vi "System.vi"() -> ()   [LabVIEW 2020]
doc: "Use this template to build a producer/consumer design pattern with events to produce queue items. Use this design pattern instead of the User Interface Event Handler pattern for user interfaces when you want to execute code asynchronously in response to an event without slowing the user interface responsiveness."
uses:
  <vilib>/Instr/_visa.llb/VISA Configure Serial Port (Instr).vi
panel:
  in  "Initialize":bool
  out "Geneator Torque":dbl(knob) scale=0.0..10.0
  out "Generator Speed":dbl(knob) scale=0.0..100.0
  out "Motor Speed":dbl(knob) scale=0.0..100.0
  out "Motor Torque":dbl(knob) scale=0.0..10.0
  out "Motor Load":dbl(slide) scale=0.0..10.0
  out "PWM":dbl
  out "Data Read":string
  in  "Baud rate (9600)":u32=9600
  in  "Write Data":bool
  in  "Data PostFix":string
  in  "VISA resource name":refnum<visa-resource-name>
  in  "Close":bool
  in  "Open":bool
  out "Connected":bool
  in  "stop":bool
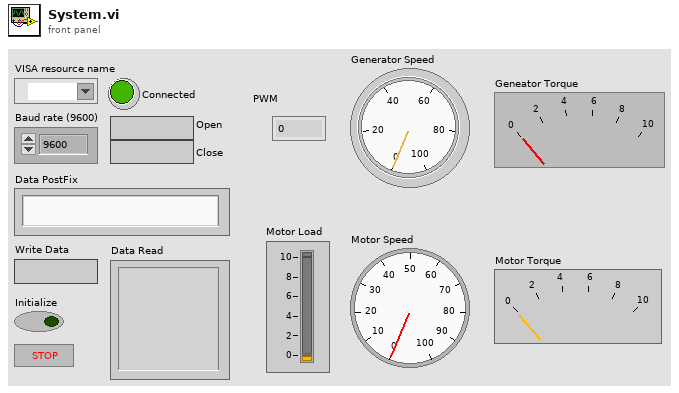
[diagram p1: front panel]
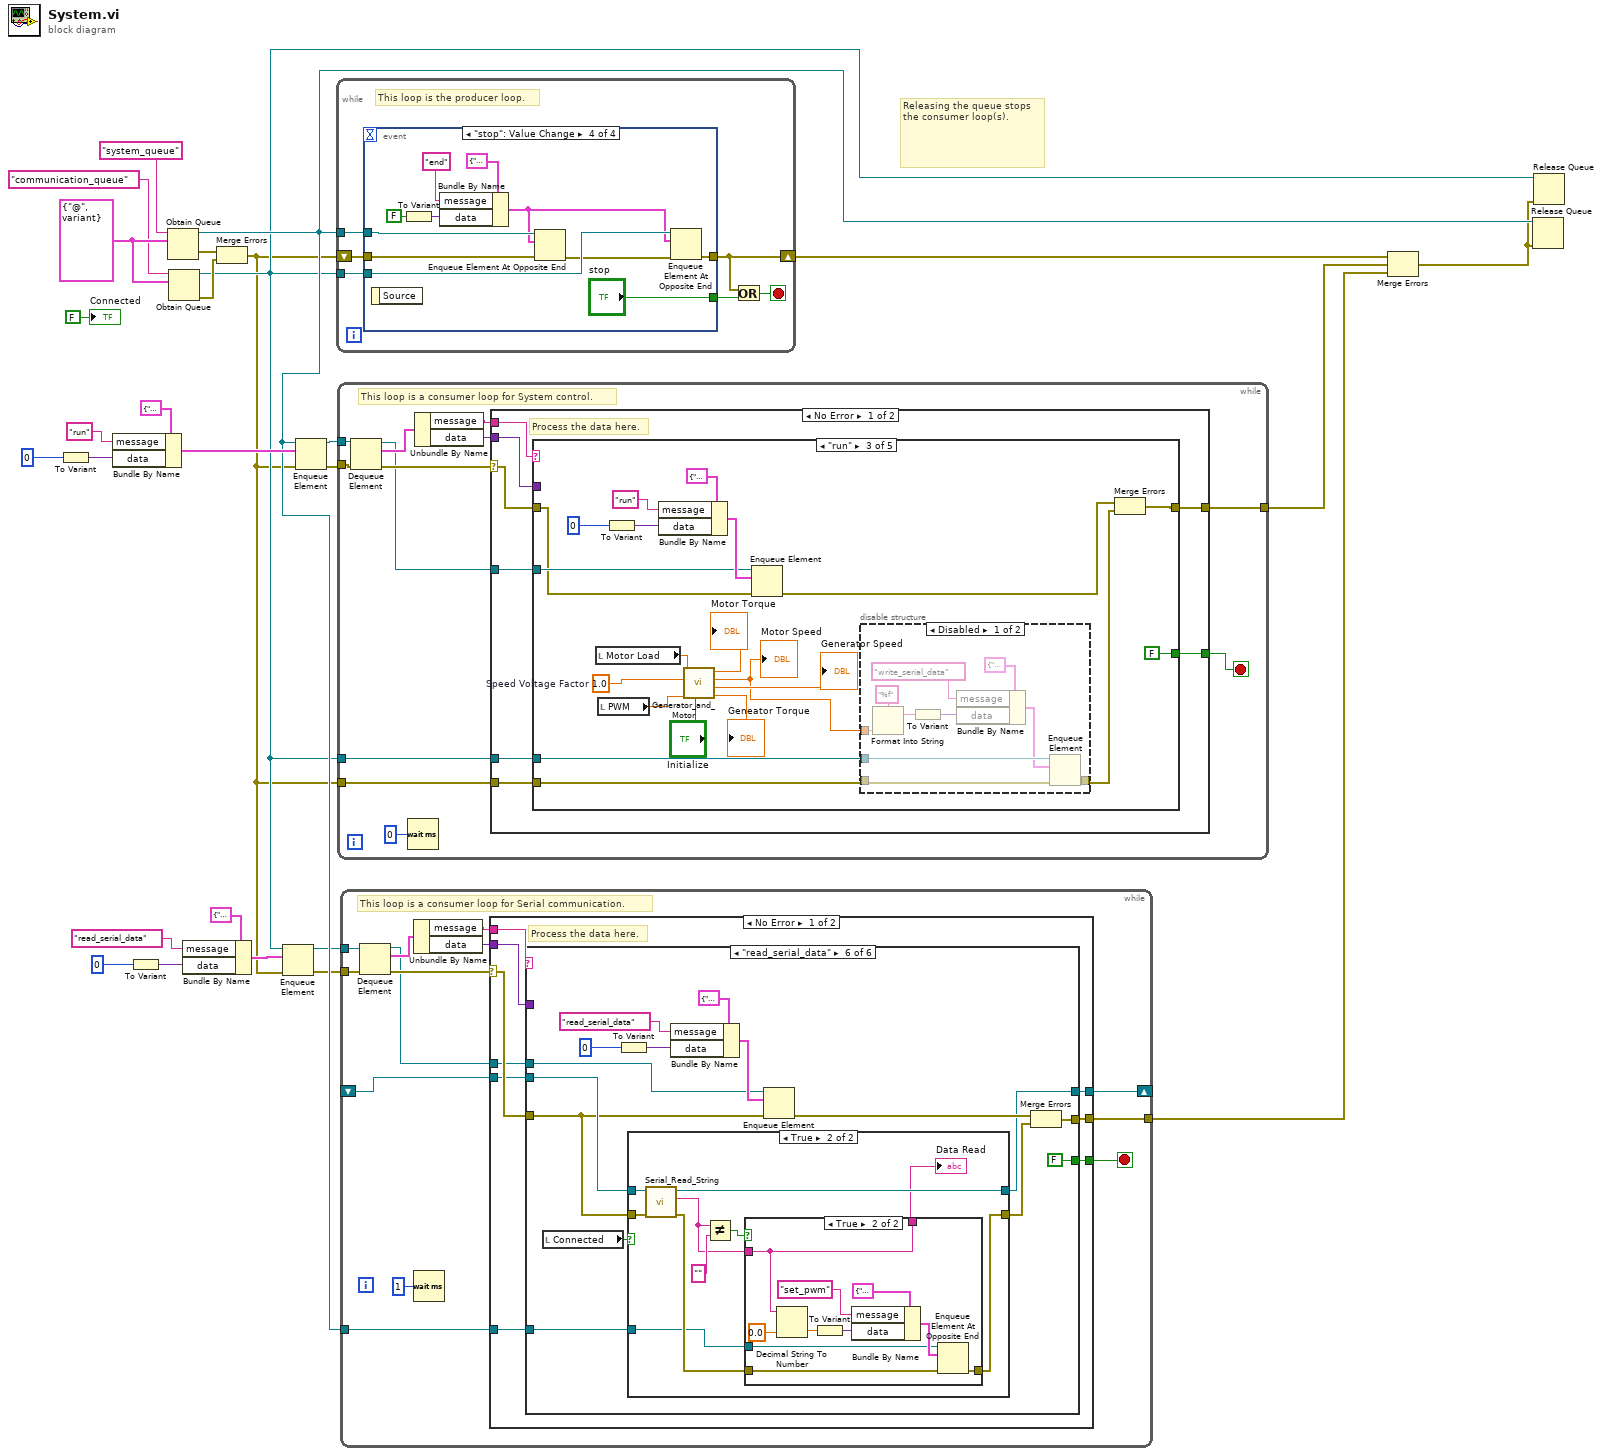
[diagram p0: block diagram]
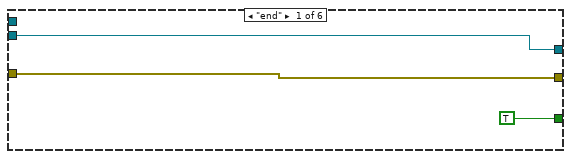
[diagram p2: hidden frame]
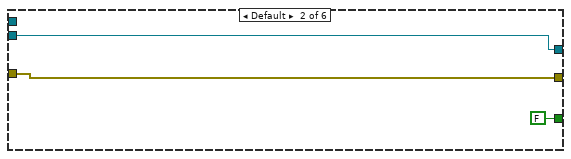
[diagram p3: hidden frame]
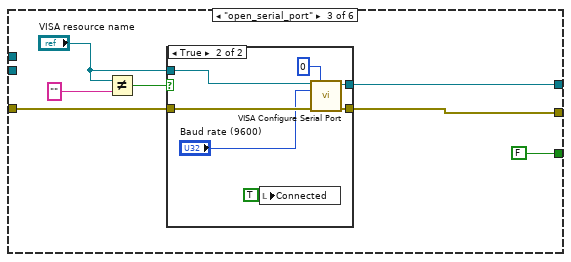
[diagram p4: hidden frame]
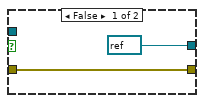
[diagram p5: hidden frame]
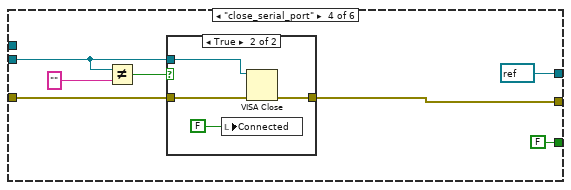
[diagram p6: hidden frame]
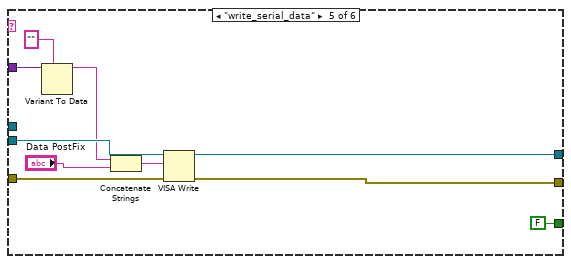
[diagram p8: hidden frame]
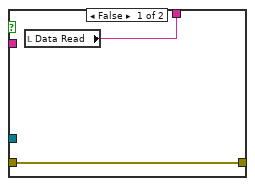
[diagram p10: hidden frame]
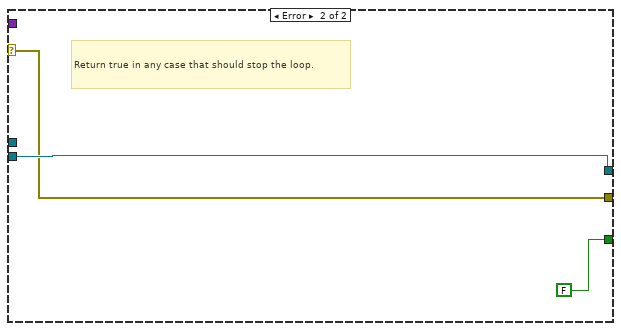
[diagram p11: hidden frame]
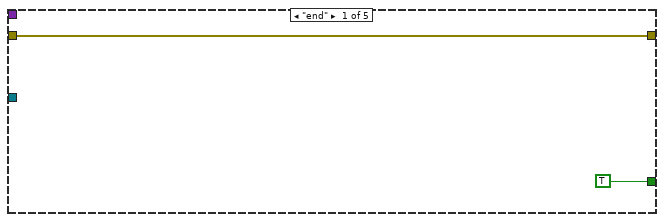
[diagram p12: hidden frame]
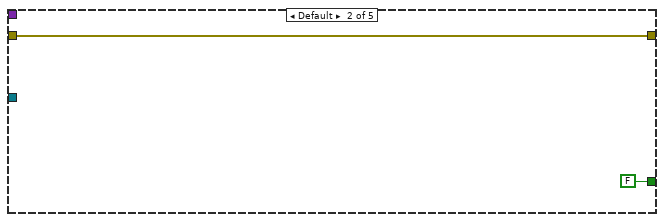
[diagram p13: hidden frame]
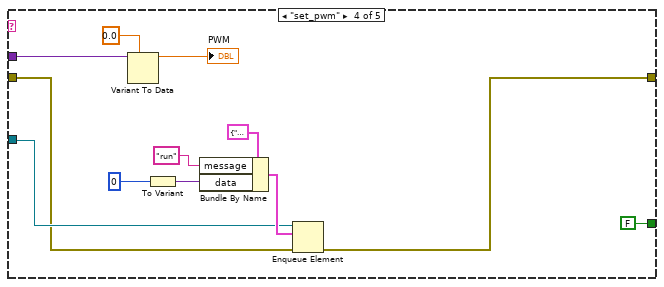
[diagram p15: hidden frame]
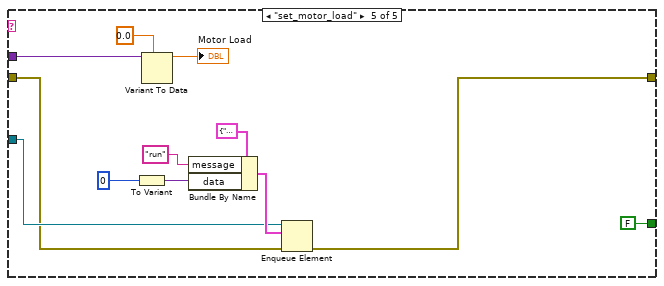
[diagram p16: hidden frame]
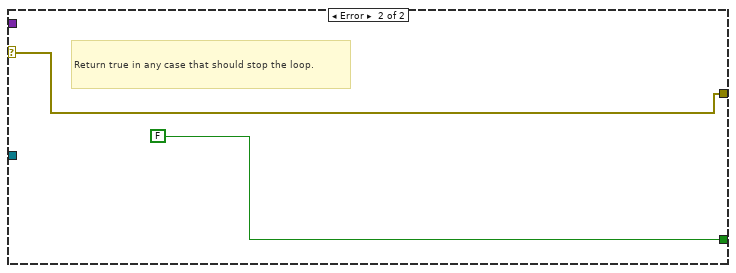
[diagram p17: hidden frame]
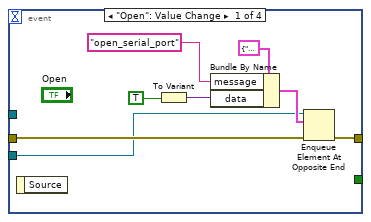
[diagram p18: hidden frame]
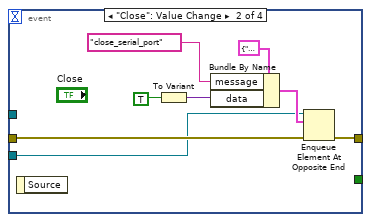
[diagram p19: hidden frame]
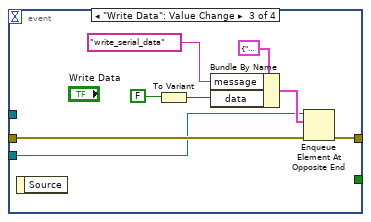
[diagram p20: hidden frame]
diagram:
  w26 = cluster{"message":string, "data":variant} {"message"="@", "data"=variant}
  # "Releasing the queue stops the consumer loop(s)."
  n1 = To Variant(anything=0) -> (Variant=w20:variant)
  n2 = Bundle By Name(cluster=cluster{"message":string, "data":variant} {"message"="@", "data"=variant}, "message"="run", "data"=w20) -> (w23:cluster{"message":string, "data":variant})
  n3 = To Variant(anything=0) -> (Variant=w8:variant)
  n4 = Obtain Queue(name (unnamed)="system_queue", element data type=w26) -> (queue out=w17:refnum<queue>, error out=w25:errorcluster)  [unwired: 3 in, 1 out]
  n5 = Obtain Queue(name (unnamed)="communication_queue", element data type=w26) -> (queue out=w2:refnum<queue>, error out=w24:errorcluster)  [unwired: 3 in, 1 out]
  n6 = Bundle By Name(cluster=cluster{"message":string, "data":variant} {"message"="@", "data"=variant}, "message"="read_serial_data", "data"=w8) -> (w11:cluster{"message":string, "data":variant})
  n7 = Merge Errors(w25, w24) -> (w1:errorcluster)
  n8 = Enqueue Element(queue=w2, element=w11, error in (no error)=w1) -> (queue out=w5:refnum<queue>, error out=w6:errorcluster)  [unwired: 1 in, 1 out]
  n9 = Enqueue Element(queue=w17, element=w23, error in (no error)=w1) -> (queue out=w16:refnum<queue>, error out=w18:errorcluster)  [unwired: 1 in, 1 out]
  n10 = while {
    shift-right: [w29] -> w13
    shift-left: w1 -> [w32]
    tunnel: w17 -> [w33]
    tunnel: w2 -> [w28]
    stop <- w30 stop-if-true
    # "This loop is the producer loop."
    n11 = event shown="[3] \"stop\": Value Change" {
      selector: _ -> [_ _ _ _]
      dyn-events: _ -> [_ _ _ _]
      timeout: _ -> [_ _ _ _]
      tunnel: w33 -> [_ _ _ w62]
      tunnel: w32 -> [w37 w45 w53 w61]
      tunnel: [w36 w44 w52 w65] -> w29
      tunnel: [_ _ _ "stop"] -> w31
      tunnel: w28 -> [w35 w43 w51 w64]
      event "Open": Value Change {
        n12 = event-data() -> ()  [unwired: 1 in, 1 out]
        n13 = To Variant(anything=TRUE ("Open")) -> (Variant=w38:variant)
        n14 = Bundle By Name(cluster=cluster{"message":string, "data":variant} {"message"="@", "data"=variant}, "message"="open_serial_port", "data"=w38) -> (w41:cluster{"message":string, "data":variant})
        n15 = Enqueue Element At Opposite End(queue=w35, element=w41, error in (no error)=w37) -> (error out=w36:errorcluster)  [unwired: 1 in, 2 out]
      }
      event "Close": Value Change {
        n16 = event-data() -> ()  [unwired: 1 in, 1 out]
        n17 = To Variant(anything=TRUE ("Close")) -> (Variant=w46:variant)
        n18 = Bundle By Name(cluster=cluster{"message":string, "data":variant} {"message"="@", "data"=variant}, "message"="close_serial_port", "data"=w46) -> (w49:cluster{"message":string, "data":variant})
        n19 = Enqueue Element At Opposite End(queue=w43, element=w49, error in (no error)=w45) -> (error out=w44:errorcluster)  [unwired: 1 in, 2 out]
      }
      event "Write Data": Value Change {
        n20 = event-data() -> ()  [unwired: 1 in, 1 out]
        n21 = To Variant(anything=FALSE ("Write Data")) -> (Variant=w54:variant)
        n22 = Bundle By Name(cluster=cluster{"message":string, "data":variant} {"message"="@", "data"=variant}, "message"="write_serial_data", "data"=w54) -> (w57:cluster{"message":string, "data":variant})
        n23 = Enqueue Element At Opposite End(queue=w51, element=w57, error in (no error)=w53) -> (error out=w52:errorcluster)  [unwired: 1 in, 2 out]
      }
      event "stop": Value Change {
        n24 = event-data() -> ()  [unwired: 1 in, 1 out]
        n25 = To Variant(anything=FALSE ("stop")) -> (Variant=w66:variant)
        n26 = Bundle By Name(cluster=cluster{"message":string, "data":variant} {"message"="@", "data"=variant}, "message"="end", "data"=w66) -> (w59:cluster{"message":string, "data":variant})
        n27 = Enqueue Element At Opposite End(queue=w62, element=w59, error in (no error)=w61) -> (error out=w60:errorcluster)  [unwired: 1 in, 2 out]
        n28 = Enqueue Element At Opposite End(queue=w64, element=w59, error in (no error)=w60) -> (error out=w65:errorcluster)  [unwired: 1 in, 2 out]
      }
    }
    n29 = Or(x=w29, y=w31) -> (x .or. y?=w30:bool)
  }
  n30 = while {
    tunnel: w16 -> [w80]
    tunnel: w18 -> [w76]
    tunnel: [w71] -> w12
    tunnel: w2 -> [w70]
    tunnel: w1 -> [w69]
    stop <- w78 stop-if-true
    # "This loop is a consumer loop for System control."
    n31 = Dequeue Element(queue=w80, error in (no error)=w76) -> (queue out=w73:refnum<queue>, element=w77:cluster{"message":string, "data":variant}, error out=w79:errorcluster)  [unwired: 1 in, 1 out]
    n32 = Wait (ms)(milliseconds to wait=u32 0) -> ()  [unwired: 1 out]
    n33 = Unbundle By Name(w77) -> ("message"=w72:string, "data"=w75:variant)
    n34 = case shown="No Error" w79 {
      selector: w79 -> [w86 w148]
      tunnel: [w84 FALSE] -> w78
      tunnel: w72 -> [w88 _]
      tunnel: w75 -> [w87 _]
      tunnel: w73 -> [w85 _]
      tunnel: [w83 w148] -> w71
      tunnel: w70 -> [w82 _]
      tunnel: w69 -> [w81 _]
      frame No Error {
        # "Process the data here."
        n35 = case shown="\"run\"" w88 {
          tunnel: w87 -> [_ _ _ w135 w145]
          tunnel: w86 -> [w89 w91 w107 w126 w138]
          tunnel: w85 -> [_ _ w108 w127 w139]
          tunnel: [TRUE FALSE FALSE FALSE FALSE] -> w84
          tunnel: [w89 w91 w96 w124 w136] -> w83
          tunnel: w82 -> [_ _ w98 _ _]
          tunnel: w81 -> [_ _ w97 _ _]
          frame "end" {
          }
          frame Default {
          }
          frame "run" {
            w104 = 1.0  # Speed Voltage Factor
            n36 = local read "Motor Load"() -> (w105:dbl)
            n37 = local read "PWM"() -> (w106:dbl)
            n38 = To Variant(anything=0) -> (Variant=w110:variant)
            n39 = Bundle By Name(cluster=cluster{"message":string, "data":variant} {"message"="@", "data"=variant}, "message"="run", "data"=w110) -> (w113:cluster{"message":string, "data":variant})
            n40 = call "Generator_and_Motor.vi"("Initialize"="Initialize", "PWM"=w106, "Speed Voltage Factor"=w104, "Motor Load"=w105) -> ("Geneator Torque"=→"Geneator Torque":dbl, "Generator Speed"=→"Generator Speed":dbl, "Motor Speed"=w93:dbl, "Motor Torque"=→"Motor Torque":dbl)  [unwired: 4 in]
            "Motor Speed" <- w93
            n41 = Enqueue Element(queue=w108, element=w113, error in (no error)=w107) -> (error out=w95:errorcluster)  [unwired: 1 in, 2 out]
            n42 = disable-structure shown="Disabled" {
              disable-tunnel: w98 -> [w123 _]
              disable-tunnel: w97 -> [w122 _]
              disable-tunnel: [w121 _] -> w94
              disable-tunnel: w93 -> [w120 _]
              frame Disabled {
                n43 = Format Into String(format string="%f", w120) -> (resulting string=w115:string)  [unwired: 2 in, 1 out]
                n44 = To Variant(anything=w115) -> (Variant=w119:variant)
                n45 = Bundle By Name(cluster=cluster{"message":string, "data":variant} {"message"="@", "data"=variant}, "message"="write_serial_data", "data"=w119) -> (w116:cluster{"message":string, "data":variant})
                n46 = Enqueue Element(queue=w123, element=w116, error in (no error)=w122) -> (error out=w121:errorcluster)  [unwired: 1 in, 2 out]
              }
              frame Enabled {
              }
            }
            n47 = Merge Errors(w95, w94) -> (w96:errorcluster)
          }
          frame "set_pwm" {
            n48 = Variant To Data(type=0.0, Variant=w135) -> (data=→"PWM":dbl)  [unwired: 1 in, 1 out]
            n49 = To Variant(anything=0) -> (Variant=w129:variant)
            n50 = Bundle By Name(cluster=cluster{"message":string, "data":variant} {"message"="@", "data"=variant}, "message"="run", "data"=w129) -> (w132:cluster{"message":string, "data":variant})
            n51 = Enqueue Element(queue=w127, element=w132, error in (no error)=w126) -> (error out=w124:errorcluster)  [unwired: 1 in, 2 out]
          }
          frame "set_motor_load" {
            n52 = To Variant(anything=0) -> (Variant=w141:variant)
            n53 = Variant To Data(type=0.0, Variant=w145) -> (data=→"Motor Load":dbl)  [unwired: 1 in, 1 out]
            n54 = Bundle By Name(cluster=cluster{"message":string, "data":variant} {"message"="@", "data"=variant}, "message"="run", "data"=w141) -> (w144:cluster{"message":string, "data":variant})
            n55 = Enqueue Element(queue=w139, element=w144, error in (no error)=w138) -> (error out=w136:errorcluster)  [unwired: 1 in, 2 out]
          }
        }
      }
      frame Error {
        # "Return true in any case that should stop the loop."
      }
    }
  }
  n56 = while {
    tunnel: w5 -> [w162]
    tunnel: w6 -> [w158]
    shift-right: [w155] -> _
    shift-left: _ -> [w154]
    tunnel: [w153] -> w4
    tunnel: w17 -> [w150]
    stop <- w160 stop-if-true
    # "This loop is a consumer loop for Serial communication."
    n57 = Dequeue Element(queue=w162, error in (no error)=w158) -> (queue out=w152:refnum<queue>, element=w159:cluster{"message":string, "data":variant}, error out=w161:errorcluster)  [unwired: 1 in, 1 out]
    n58 = Unbundle By Name(w159) -> ("message"=w157:string, "data"=w156:variant)
    n59 = Wait (ms)(milliseconds to wait=u32 1) -> ()  [unwired: 1 out]
    n60 = case shown="No Error" w161 {
      selector: w161 -> [w169 w255]
      tunnel: [w163 FALSE] -> w160
      tunnel: w157 -> [w171 _]
      tunnel: w156 -> [w170 _]
      tunnel: [w168 w256] -> w155
      tunnel: w154 -> [w167 w256]
      tunnel: [w166 w255] -> w153
      tunnel: w152 -> [w165 _]
      tunnel: w150 -> [w164 _]
      frame No Error {
        # "Process the data here."
        n61 = case shown="\"read_serial_data\"" w171 {
          tunnel: w170 -> [_ _ _ _ w209 _]
          tunnel: w169 -> [w173 w176 w184 w200 w214 w223]
          tunnel: [w174 w177 w180 refnum<visa-resource-name> refnum ("VISA resource name out") w213 w219] -> w168
          tunnel: w167 -> [w174 w177 _ w197 w215 w224]
          tunnel: [w173 w176 w179 w196 w212 w220] -> w166
          tunnel: w165 -> [_ _ _ _ _ w226]
          tunnel: w164 -> [_ _ _ _ _ w217]
          tunnel: [TRUE FALSE FALSE FALSE FALSE FALSE] -> w163
          frame "end" {
          }
          frame Default {
          }
          frame "open_serial_port" {
            n62 = Not Equal?(x="VISA resource name", y="") -> (x != y?=w182:bool)
            n63 = case shown="True" w182 {
              tunnel: w184 -> [w185 w192]
              tunnel: "VISA resource name" -> [_ w189]
              tunnel: [refnum<visa-resource-name> refnum ("VISA resource name") w190] -> w180
              tunnel: [w185 w191] -> w179
              frame False {
              }
              frame True {
                n64 = local write "Connected"(TRUE ("Boolean")) -> ()
                n65 = call-poly "VISA Configure Serial Port"("VISA resource name"=w189, "timeout (10sec)"=u32 0, "baud rate (9600)"="Baud rate (9600)", "error in (no error)"=w192) -> ("VISA resource name out"=w190:refnum<visa-resource-name>, "error out"=w191:errorcluster)  [unwired: 10 in]
              }
            }
          }
          frame "close_serial_port" {
            n66 = Not Equal?(x=w197, y="") -> (x != y?=w198:bool)
            n67 = case shown="True" w198 {
              tunnel: w200 -> [w201 w205]
              tunnel: w197 -> [_ w204]
              tunnel: [w201 w202] -> w196
              frame False {
              }
              frame True {
                n68 = local write "Connected"(FALSE ("Boolean")) -> ()
                n69 = VISA Close(VISA resource name=w204, error in (no error)=w205) -> (error out=w202:errorcluster)
              }
            }
          }
          frame "write_serial_data" {
            n70 = Variant To Data(type="" ("Data PostFix"), Variant=w209) -> (data=w207:string)  [unwired: 1 in, 1 out]
            n71 = Concatenate Strings(w207, "Data PostFix") -> (w208:string)
            n72 = VISA Write(VISA resource name=w215, write buffer=w208, error in (no error)=w214) -> (VISA resource name out=w213:refnum<visa-resource-name>, error out=w212:errorcluster)  [unwired: 1 out]
          }
          frame "read_serial_data" {
            n73 = local read "Connected"() -> (w218:bool)
            n74 = To Variant(anything=0) -> (Variant=w227:variant)
            n75 = case shown="True" w218 {
              tunnel: w224 -> [w232 w241]
              tunnel: w223 -> [w231 w237]
              tunnel: [w231 w233] -> w221
              tunnel: [w232 w242] -> w219
              tunnel: w217 -> [_ w234]
              frame False {
              }
              frame True {
                n76 = call "Serial_Read_String.vi"("error in (no error)"=w237, "VISA Refnum in"=w241) -> ("error out"=w235:errorcluster, "read buffer"=w238:string, "VISA Refnum out"=w242:refnum<visa-resource-name>)  [unwired: 7 in]
                n77 = Not Equal?(x=w238, y="") -> (x != y?=w239:bool)
                n78 = case shown="True" w239 {
                  tunnel: [w244 w246] -> w236
                  tunnel: w238 -> [_ w246]
                  tunnel: w235 -> [w243 w248]
                  tunnel: w234 -> [_ w247]
                  tunnel: [w243 w245] -> w233
                  frame False {
                    n79 = local read "Data Read"() -> (w244:string)
                  }
                  frame True {
                    n80 = Decimal String To Number(string=w246, default (0L)=0.0 ("default (0 I32)")) -> (number=w250:dbl)  [unwired: 1 in, 1 out]
                    n81 = To Variant(anything=w250) -> (Variant=w254:variant)
                    n82 = Bundle By Name(cluster=cluster{"message":string, "data":variant} {"message"="@", "data"=variant}, "message"="set_pwm", "data"=w254) -> (w253:cluster{"message":string, "data":variant})
                    n83 = Enqueue Element At Opposite End(queue=w247, element=w253, error in (no error)=w248) -> (error out=w245:errorcluster)  [unwired: 1 in, 2 out]
                  }
                }
                "Data Read" <- w236
              }
            }
            n84 = Bundle By Name(cluster=cluster{"message":string, "data":variant} {"message"="@", "data"=variant}, "message"="read_serial_data", "data"=w227) -> (w230:cluster{"message":string, "data":variant})
            n85 = Enqueue Element(queue=w226, element=w230, error in (no error)=w223) -> (error out=w222:errorcluster)  [unwired: 1 in, 2 out]
            n86 = Merge Errors(w222, w221) -> (w220:errorcluster)
          }
        }
      }
      frame Error {
        # "Return true in any case that should stop the loop."
      }
    }
  }
  n87 = Merge Errors(w13, w12, w4) -> (w3:errorcluster)
  n88 = Release Queue(queue=w17, error in (no error)=w3) -> ()  [unwired: 1 in, 3 out]
  n89 = Release Queue(queue=w2, error in (no error)=w3) -> ()  [unwired: 1 in, 3 out]
  "Connected" <- FALSE ("Boolean")
